vi "CISS Data.vi"() -> (2 "B array 1":dbl[](array[numeric])=[-14.0, -13.8, -13.6, -13.4, -13.2, -13.0, -12.8, -12.6, -12.4, -12.2, -12.0, -11.8, -11.6, -11.4, -11.2, -11.0, -10.8, -10.6, -10.4, -10.2, -10.0, -9.8, -9.6, -9.399999999999999, -9.2, -9.0, -8.8, -8.6, -8.399999999999999, -8.2, -8.0, -7.8, -7.6, -7.3999999999999995, -7.199999999999999, -7.0, -6.8, -6.6, -6.3999999999999995, -6.199999999999999, -6.0, -5.799999999999999, -5.6, -5.4, -5.199999999999999, -5.0, -4.799999999999999, -4.6, -4.399999999999999, -4.199999999999999, -4.0, -3.799999999999999, -3.5999999999999996, -3.3999999999999986, -3.1999999999999993, -3.0, -2.799999999999999, -2.5999999999999996, -2.3999999999999986, -2.1999999999999993, -2.0, -1.799999999999999, -1.5999999999999996, -1.3999999999999986, -1.1999999999999993, -1.0, -0.7999999999999989, -0.5999999999999996, -0.3999999999999986, -0.1999999999999993, 0.0, 0.20000000000000107, 0.40000000000000036, 0.6000000000000014, 0.8000000000000007, 1.0, 1.200000000000001, 1.4000000000000004, 1.6000000000000014, 1.8000000000000007, 2.0, 2.1999999999999993, 2.400000000000002, 2.6000000000000014, 2.8000000000000007, 3.0, 3.1999999999999993, 3.400000000000002, 3.6000000000000014, 3.8000000000000007, 4.0, 4.199999999999999, 4.400000000000002, 4.600000000000001, 4.800000000000001, 5.0, 5.200000000000003, 5.400000000000002, 5.600000000000001, 5.800000000000001, 6.0, 6.200000000000003, 6.400000000000002, 6.600000000000001, 6.800000000000001, 7.0, 7.200000000000003, 7.400000000000002, 7.600000000000001, 7.800000000000001, 8.0, 8.200000000000003, 8.400000000000002, 8.600000000000001, 8.8, 9.0, 9.200000000000003, 9.400000000000002, 9.600000000000001, 9.8, 10.0, 10.200000000000003, 10.400000000000002, 10.600000000000001, 10.8, 11.0, 11.200000000000003, 11.400000000000002, 11.600000000000001, 11.8, 12.0, 12.200000000000003, 12.400000000000002, 12.600000000000001, 12.8, 13.0, 13.200000000000003, 13.400000000000002, 13.600000000000001, 13.8, 14.0], 3 "G vs X":cluster{dbl[], dbl[]}[](array[cluster]))   [LabVIEW 2019]
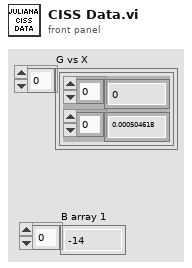
[diagram p1: front panel]
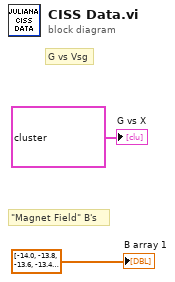
[diagram p0: block diagram]
diagram:
  # "G vs Vsg"
  # "\"Magnet Field\" B's"
  "B array 1" <- dbl[] [-14.0, -13.8, -13.6, -13.4, -13.2, -13.0, -12.8, -12.6, -12.4, -12.2, -12.0, -11.8, -11.6, -11.4, -11.2, -11.0, -10.8, -10.6, -10.4, -10.2, -10.0, -9.8, -9.6, -9.399999999999999, -9.2, -9.0, -8.8, -8.6, -8.399999999999999, -8.2, -8.0, -7.8, -7.6, -7.3999999999999995, -7.199999999999999, -7.0, -6.8, -6.6, -6.3999999999999995, -6.199999999999999, -6.0, -5.799999999999999, -5.6, -5.4, -5.199999999999999, -5.0, -4.799999999999999, -4.6, -4.399999999999999, -4.199999999999999, -4.0, -3.799999999999999, -3.5999999999999996, -3.3999999999999986, -3.1999999999999993, -3.0, -2.799999999999999, -2.5999999999999996, -2.3999999999999986, -2.1999999999999993, -2.0, -1.799999999999999, -1.5999999999999996, -1.3999999999999986, -1.1999999999999993, -1.0, -0.7999999999999989, -0.5999999999999996, -0.3999999999999986, -0.1999999999999993, 0.0, 0.20000000000000107, 0.40000000000000036, 0.6000000000000014, 0.8000000000000007, 1.0, 1.200000000000001, 1.4000000000000004, 1.6000000000000014, 1.8000000000000007, 2.0, 2.1999999999999993, 2.400000000000002, 2.6000000000000014, 2.8000000000000007, 3.0, 3.1999999999999993, 3.400000000000002, 3.6000000000000014, 3.8000000000000007, 4.0, 4.199999999999999, 4.400000000000002, 4.600000000000001, 4.800000000000001, 5.0, 5.200000000000003, 5.400000000000002, 5.600000000000001, 5.800000000000001, 6.0, 6.200000000000003, 6.400000000000002, 6.600000000000001, 6.800000000000001, 7.0, 7.200000000000003, 7.400000000000002, 7.600000000000001, 7.800000000000001, 8.0, 8.200000000000003, 8.400000000000002, 8.600000000000001, 8.8, 9.0, 9.200000000000003, 9.400000000000002, 9.600000000000001, 9.8, 10.0, 10.200000000000003, 10.400000000000002, 10.600000000000001, 10.8, 11.0, 11.200000000000003, 11.400000000000002, 11.600000000000001, 11.8, 12.0, 12.200000000000003, 12.400000000000002, 12.600000000000001, 12.8, 13.0, 13.200000000000003, 13.400000000000002, 13.600000000000001, 13.8, 14.0] ("Array")
  "G vs X" <- cluster{dbl[], dbl[]}[] [{array[977 elements], array[977 elements]}, {array[977 elements], array[977 elements]}, {array[977 elements], array[977 elements]}, {array[977 elements], array[977 elements]}, {array[977 elements], array[977 elements]}, {array[977 elements], array[977 elements]}, {array[977 elements], array[977 elements]}, {array[977 elements], array[977 elements]}, {array[977 elements], array[977 elements]}, {array[977 elements], array[977 elements]}, {array[977 elements], array[977 elements]}, {array[977 elements], array[977 elements]}, {array[977 elements], array[977 elements]}, {array[977 elements], array[977 elements]}, {array[977 elements], array[977 elements]}, {array[977 elements], array[977 elements]}, {array[977 elements], array[977 elements]}, {array[977 elements], array[977 elements]}, {array[977 elements], array[977 elements]}, {array[977 elements], array[977 elements]}, {array[977 elements], array[977 elements]}, {array[977 elements], array[977 elements]}, {array[977 elements], array[977 elements]}, {array[977 elements], array[977 elements]}, {array[977 elements], array[977 elements]}, {array[977 elements], array[977 elements]}, {array[977 elements], array[977 elements]}, {array[977 elements], array[977 elements]}, {array[977 elements], array[977 elements]}, {array[977 elements], array[977 elements]}, {array[977 elements], array[977 elements]}, {array[977 elements], array[977 elements]}, {array[977 elements], array[977 elements]}, {array[977 elements], array[977 elements]}, {array[977 elements], array[977 elements]}, {array[977 elements], array[977 elements]}, {array[977 elements], array[977 elements]}, {array[977 elements], array[977 elements]}, {array[977 elements], array[977 elements]}, {array[977 elements], array[977 elements]}, {array[977 elements], array[977 elements]}, {array[977 elements], array[977 elements]}, {array[977 elements], array[977 elements]}, {array[977 elements], array[977 elements]}, {array[977 elements], array[977 elements]}, {array[977 elements], array[977 elements]}, {array[977 elements], array[977 elements]}, {array[977 elements], array[977 elements]}, {array[977 elements], array[977 elements]}, {array[977 elements], array[977 elements]}, {array[977 elements], array[977 elements]}, {array[977 elements], array[977 elements]}, {array[977 elements], array[977 elements]}, {array[977 elements], array[977 elements]}, {array[977 elements], array[977 elements]}, {array[977 elements], array[977 elements]}, {array[977 elements], array[977 elements]}, {array[977 elements], array[977 elements]}, {array[977 elements], array[977 elements]}, {array[977 elements], array[977 elements]}, {array[977 elements], array[977 elements]}, {array[977 elements], array[977 elements]}, {array[977 elements], array[977 elements]}, {array[977 elements], array[977 elements]}, {array[977 elements], array[977 elements]}, {array[977 elements], array[977 elements]}, {array[977 elements], array[977 elements]}, {array[977 elements], array[977 elements]}, {array[977 elements], array[977 elements]}, {array[977 elements], array[977 elements]}, {array[977 elements], array[977 elements]}, {array[977 elements], array[977 elements]}, {array[977 elements], array[977 elements]}, {array[977 elements], array[977 elements]}, {array[977 elements], array[977 elements]}, {array[977 elements], array[977 elements]}, {array[977 elements], array[977 elements]}, {array[977 elements], array[977 elements]}, {array[977 elements], array[977 elements]}, {array[977 elements], array[977 elements]}, {array[977 elements], array[977 elements]}, {array[977 elements], array[977 elements]}, {array[977 elements], array[977 elements]}, {array[977 elements], array[977 elements]}, {array[977 elements], array[977 elements]}, {array[977 elements], array[977 elements]}, {array[977 elements], array[977 elements]}, {array[977 elements], array[977 elements]}, {array[977 elements], array[977 elements]}, {array[977 elements], array[977 elements]}, {array[977 elements], array[977 elements]}, {array[977 elements], array[977 elements]}, {array[977 elements], array[977 elements]}, {array[977 elements], array[977 elements]}, {array[977 elements], array[977 elements]}, {array[977 elements], array[977 elements]}, {array[977 elements], array[977 elements]}, {array[977 elements], array[977 elements]}, {array[977 elements], array[977 elements]}, {array[977 elements], array[977 elements]}, {array[977 elements], array[977 elements]}, {array[977 elements], array[977 elements]}, {array[977 elements], array[977 elements]}, {array[977 elements], array[977 elements]}, {array[977 elements], array[977 elements]}, {array[977 elements], array[977 elements]}, {array[977 elements], array[977 elements]}, {array[977 elements], array[977 elements]}, {array[977 elements], array[977 elements]}, {array[977 elements], array[977 elements]}, {array[977 elements], array[977 elements]}, {array[977 elements], array[977 elements]}, {array[977 elements], array[977 elements]}, {array[977 elements], array[977 elements]}, {array[977 elements], array[977 elements]}, {array[977 elements], array[977 elements]}, {array[977 elements], array[977 elements]}, {array[977 elements], array[977 elements]}, {array[977 elements], array[977 elements]}, {array[977 elements], array[977 elements]}, {array[977 elements], array[977 elements]}, {array[977 elements], array[977 elements]}, {array[977 elements], array[977 elements]}, {array[977 elements], array[977 elements]}, {array[977 elements], array[977 elements]}, {array[977 elements], array[977 elements]}, {array[977 elements], array[977 elements]}, {array[977 elements], array[977 elements]}, {array[977 elements], array[977 elements]}, {array[977 elements], array[977 elements]}, {array[977 elements], array[977 elements]}, {array[977 elements], array[977 elements]}, {array[977 elements], array[977 elements]}, {array[977 elements], array[977 elements]}, {array[977 elements], array[977 elements]}, {array[977 elements], array[977 elements]}, {array[977 elements], array[977 elements]}, {array[977 elements], array[977 elements]}, {array[977 elements], array[977 elements]}, {array[977 elements], array[977 elements]}, {array[977 elements], array[977 elements]}] ("G vs X")
